vi "Use Case.vi"() -> ()   [LabVIEW 2021, in "uCanDriver.lvlib" / "uCAN.lvclass"]
uses:
  uCAN.lvclass
  typedefs/frame.ctl
  typedefs/bitrates.ctl
panel:
  in  "Bitrates":T1=enum."500 kbit/s"
  in  "COM port":refnum<visa-resource-name>="COM9"
  in  "Transmit Frame":bool
  in  "New Frame":T2 {"Data" format="%.0x"}
  in  "stop":bool
  out "Received Frames":T2[](array[typedef]) {"Data" format="%.0x"}
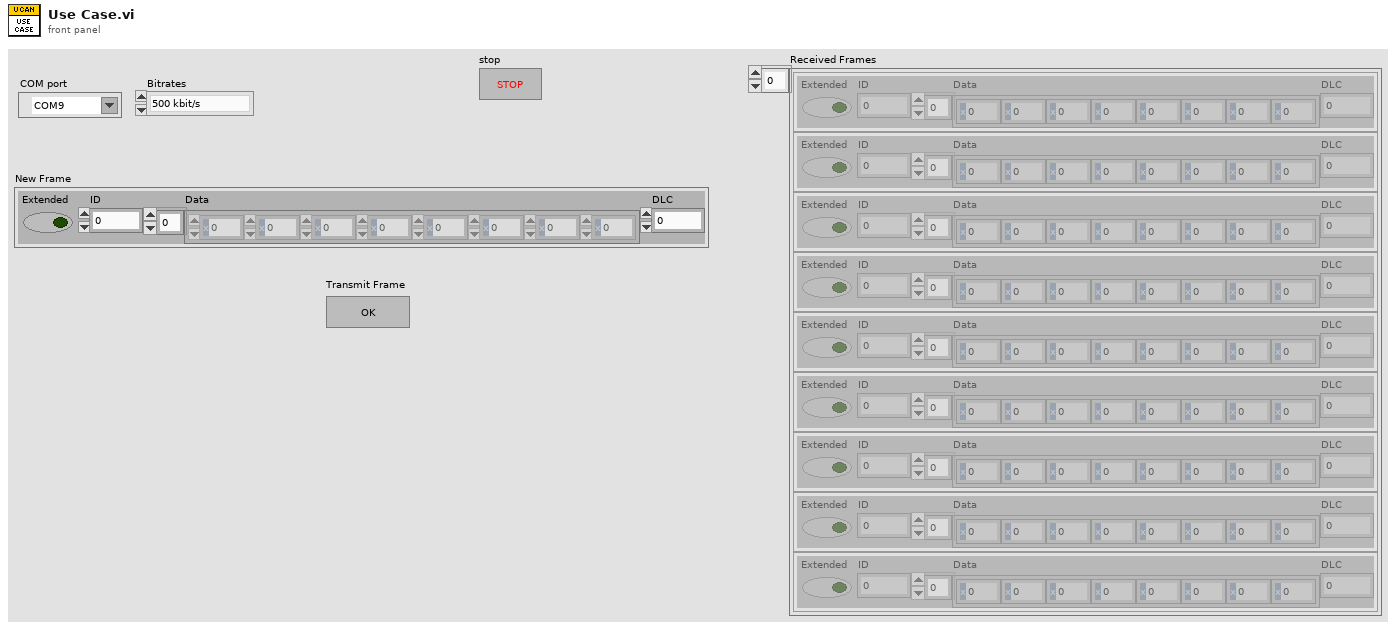
[diagram p1: front panel]
types:
  T1 = typedef "uCanDriver.lvlib/uCAN.lvclass/bitrates.ctl" = enum16{"100 kbit/s", "125 kbit/s", "250 kbit/s", "500 kbit/s", "800 kbit/s", "1 Mbit/s"}
  T2 = typedef "uCanDriver.lvlib/uCAN.lvclass/frame.ctl" = cluster{"Extended":bool, "ID":u32, "Data":u8[], "DLC":u8}
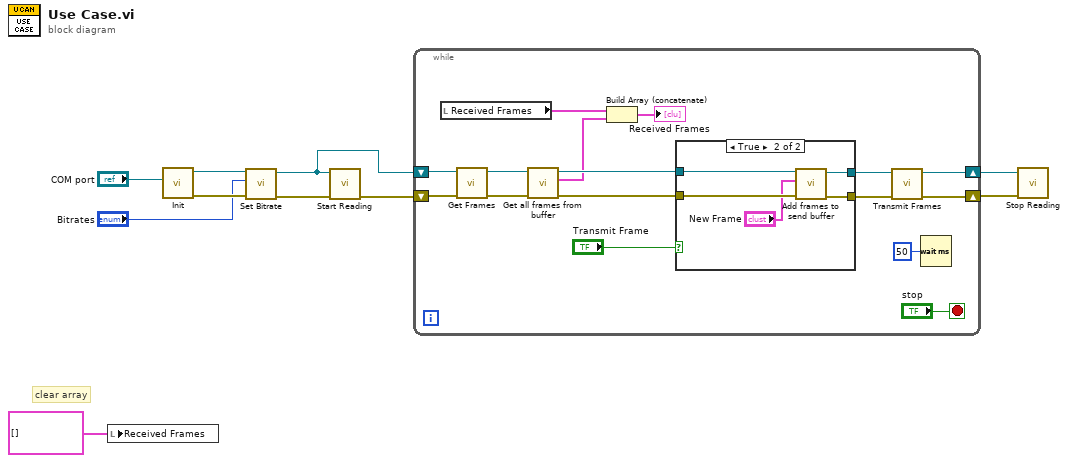
[diagram p0: block diagram]
diagram:
  # "clear array"
  n1 = local write "Received Frames"(T2[] [] ("Received Frames Array")) -> ()
  n2 = call "Init.vi"("COM port"="COM port") -> ("error out"=w8:errorcluster, "uCAN out"=w9:refnum<class "uCAN.lvclass">)  [unwired: 9 in]
  n3 = call "Set Bitrate.vi"("error in (no error)"=w8, "Bitrates"="Bitrates", "uCAN in"=w9) -> ("error out"=w6:errorcluster, "uCAN out"=w1:refnum<class "uCAN.lvclass">)  [unwired: 7 in]
  n4 = call "Start Reading.vi"("error in (no error)"=w6, "uCAN in"=w1) -> ("error out"=w2:errorcluster)  [unwired: 9 in]
  n5 = while {
    shift-right: [w12] -> w5
    shift-left: w1 -> [w26]
    shift-right: [w14] -> w4
    shift-left: w2 -> [w25]
    stop <- "stop" stop-if-true
    n6 = local read "Received Frames"() -> (w16:T2[])
    n7 = call "Get Frames.vi"("error in (no error)"=w25, "uCAN in"=w26) -> ("error out"=w24:errorcluster, "uCAN out"=w23:refnum<class "uCAN.lvclass">)  [unwired: 7 in, 1 out]
    n8 = call "Get all frames from buffer.vi"("error in (no error)"=w24, "uCAN in"=w23) -> ("error out"=w21:errorcluster, "Received Frames Array"=w15:T2[], "uCAN out"=w22:refnum<class "uCAN.lvclass">)  [unwired: 7 in]
    n9 = Build Array (concatenate)(w16, w15) -> (→"Received Frames":T2[])
    n10 = case shown="True" "Transmit Frame" {
      tunnel: w22 -> [w28 w33]
      tunnel: w21 -> [w27 w32]
      tunnel: [w27 w31] -> w20
      tunnel: [w28 w30] -> w13
      frame False {
      }
      frame True {
        n11 = call "Add frames to send buffer.vi"("error in (no error)"=w32, "New Frame"="New Frame", "uCAN in"=w33) -> ("error out"=w31:errorcluster, "uCAN out"=w30:refnum<class "uCAN.lvclass">)  [unwired: 7 in]
      }
    }
    n12 = call "Transmit Frames.vi"("error in (no error)"=w20, "uCAN in"=w13) -> ("error out"=w14:errorcluster, "uCAN out"=w12:refnum<class "uCAN.lvclass">)  [unwired: 8 in]
    n13 = Wait (ms)(milliseconds to wait=u32 50) -> ()  [unwired: 1 out]
  }
  n14 = call "Stop Reading.vi"("error in (no error)"=w4, "uCAN in"=w5) -> ()  [unwired: 8 in, 2 out]
